vi "ER2007 System Setup Panel.vi"() -> ()   [LabVIEW 2013]
uses:
  Controls/Global ER2007.vi
panel:
  in  "VPA Period":dbl=60.0 caption="(secs)" min=1.0
  in  "Log CGD Errors":bool
  in  "Barometric\nPressure":dbl=14.0 caption="(psig)" min=0.1 step=1.0 format="%.1f"
  in  "SimGalil":bool
  in  "Cell Names":string[](array[string])
  in  "PC ID":i32=1 min=1 max=2
  in  "Excel Template Path":path
  in  "NAII 2250\nWait":dbl=2.0 caption="(sec)" min=0.1 step=1.0 format="%.1f"
  in  "Generator\nON Wait":dbl=3.0 caption="(sec)" min=0.1 step=1.0 format="%.1f"
  in  "Path for Spreadsheet Files":path
  in  "Find Series Resistor\nLow Threshold Level":dbl=25.0 caption="(%)" min=0.1 format="%.1f"
  in  "PrintResData":bool
  in  "Series Resistor\nValues (Kohm)":dbl[](array[numeric])=[0.01, 0.1, 1.0, 10.0, 100.0, 1000.0]
  in  "Series Resistor High\nThreshold Level":dbl=95.0 caption="(%)" min=0.1 format="%.1f"
  in  "Series Resistor Low\nThreshold Level":dbl=10.0 caption="(%)" min=0.1 format="%.1f"
  in  "No File":bool
  in  "Agilent 33220A\nDefault Amplitude":dbl=1.0 caption="(Vrms)" min=0.1 format="%.1f"
  in  "NAII Address":string="02"
  in  "Agilent Address":string="10"
  in  "Super Password":string
  in  "User Password":string
  in  "Data File Path":path
  in  "Graph Update\nInterval":dbl=1.0 caption="(sec)" min=0.1 step=1.0 format="%.1f"
  in  "Calibration Filename":path
  in  "InvDins":bool
  in  "InvDouts":bool
  in  "SimHP":bool
  in  "SimNAI":bool
  in  "Debug":bool
  in  "Quit2LV":bool
  in  "SimDaq":bool
  out "Copyright":string="Program ER2006, Version 1.00, DCI Inc, Copyright 2006, All Rights Reserved"
  in  "Cancel":bool
  in  "OK":bool
  out "Defaults Filename":string="ER2006.dft"
  # "ER2007 System Setup Panel"
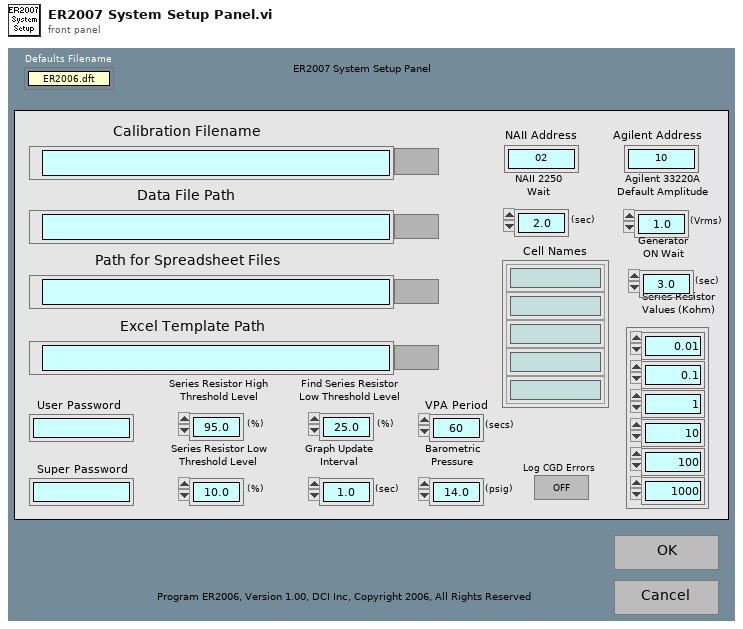
[diagram p1: front panel]
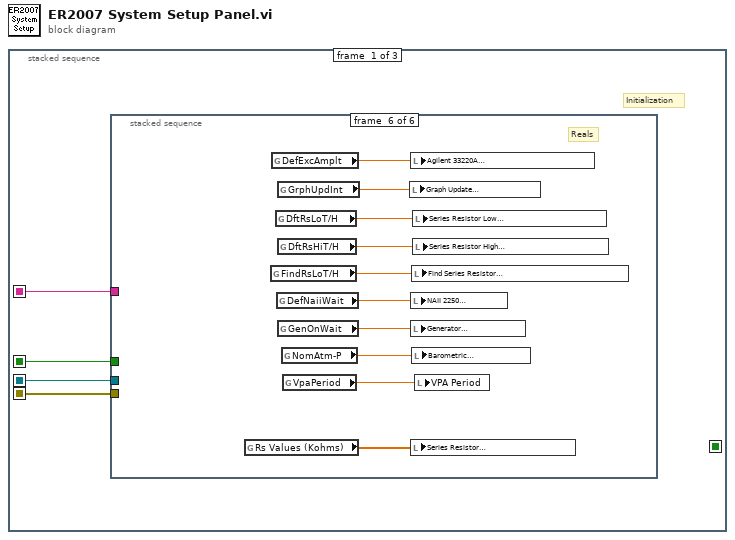
[diagram p0: block diagram]
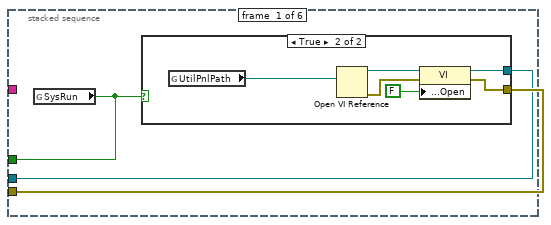
[diagram p2: hidden frame]
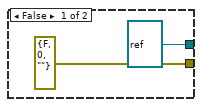
[diagram p3: hidden frame]
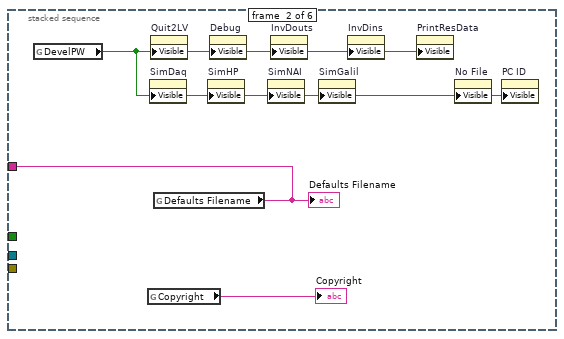
[diagram p4: hidden frame]
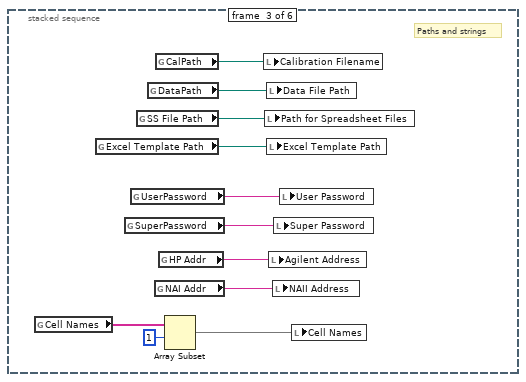
[diagram p5: hidden frame]
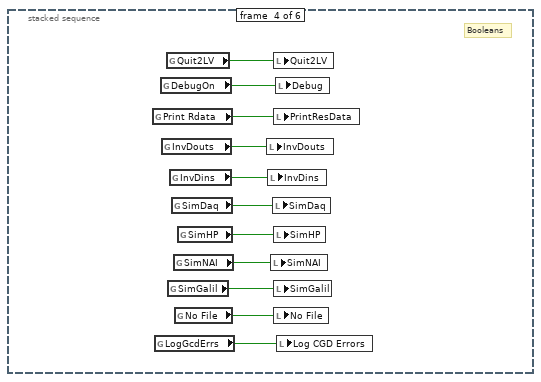
[diagram p6: hidden frame]
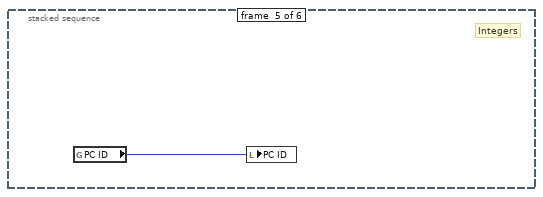
[diagram p7: hidden frame]
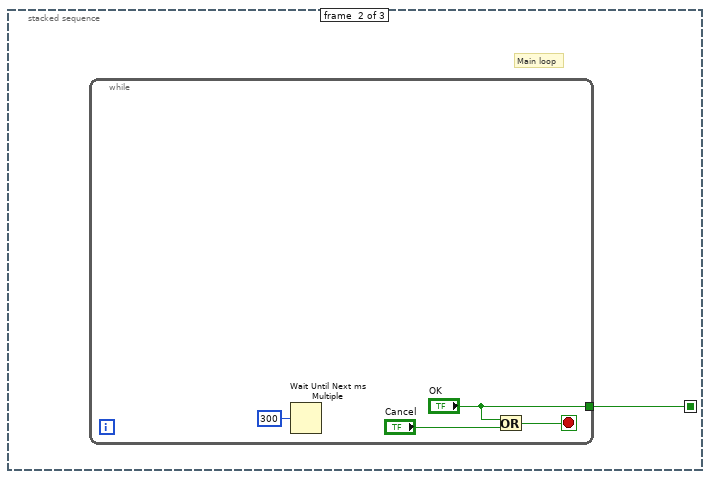
[diagram p8: hidden frame]
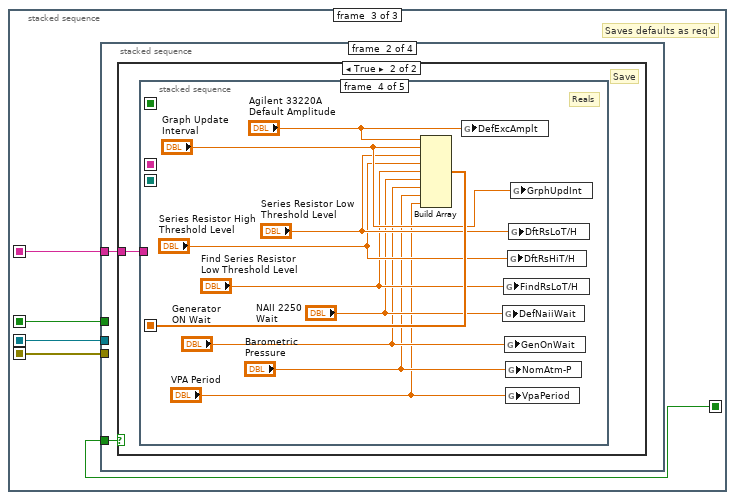
[diagram p9: hidden frame]
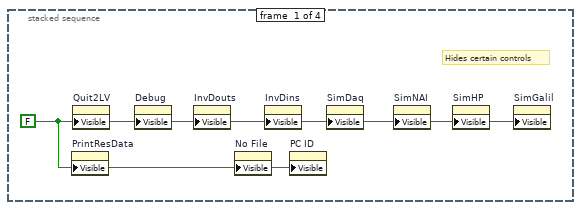
[diagram p10: hidden frame]
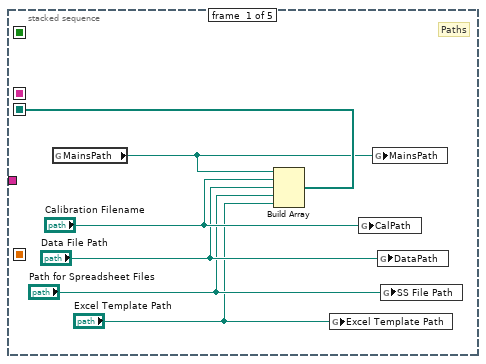
[diagram p12: hidden frame]
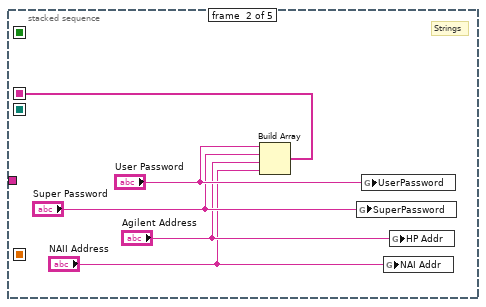
[diagram p13: hidden frame]
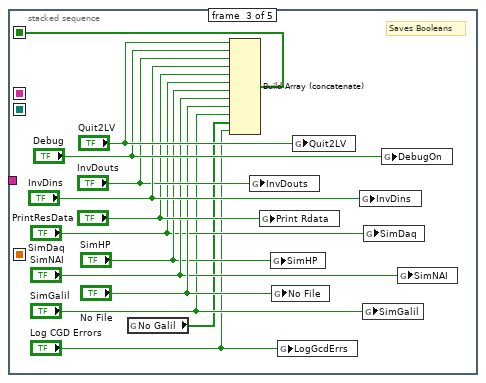
[diagram p14: hidden frame]
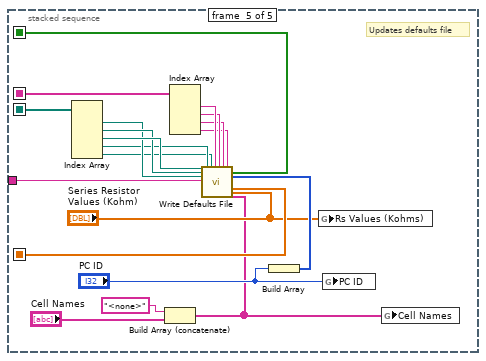
[diagram p15: hidden frame]
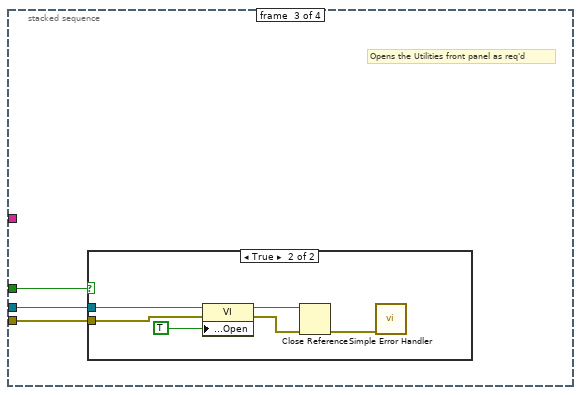
[diagram p16: hidden frame]
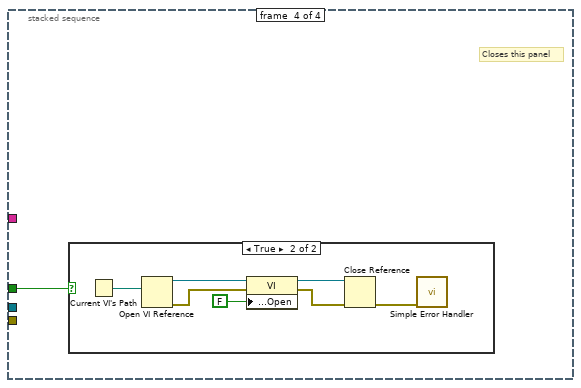
[diagram p18: hidden frame]
diagram:
  n1 = stacked-sequence {
    seq-local: [_ w52 _] -> [_ _ w61]
    seq-local: [w4 _ _] -> [_ _ w60]
    seq-local: [w3 _ _] -> [_ _ w59]
    seq-local: [w1 _ _] -> [_ _ w58]
    seq-local: [w2 _ _] -> [_ _ w57]
    frame #0 {
      # "Initialization"
      n2 = stacked-sequence {
        tunnel: [_ w18 _ _ _ _] -> w4
        tunnel: [w5 _ _ _ _ _] -> w3
        tunnel: [w7 _ _ _ _ _] -> w2
        tunnel: [w6 _ _ _ _ _] -> w1
        frame #0 {
          n3 = global read "Global ER2007.vi" "SysRun"() -> (w5:bool)
          n4 = case shown="True" w5 {
            tunnel: [refnum<vi> refnum w12] -> w6
            tunnel: [errorcluster {"status"=FALSE, "code"=0, "source"=""} ("error out") w11] -> w7
            frame False {
            }
            frame True {
              n5 = global read "Global ER2007.vi" "UtilPnlPath"() -> (w10:path)
              n6 = Open VI Reference(vi path=w10) -> (vi reference=w15:refnum<vi>, error out=w14:errorcluster)  [unwired: 5 in]
              n7 = property class="VI"(reference=w15, error in=w14, "Front Panel Window:Open"=FALSE) -> (reference out=w12:refnum<vi>, error out=w11:errorcluster)
            }
          }
        }
        frame #1 {
          n8 = global read "Global ER2007.vi" "DevelPW"() -> (w16:bool)
          n9 = global read "Global ER2007.vi" "Copyright"() -> (→"Copyright":string)
          n10 = property on="SimDaq" class="Bool (strict)"("Visible"=w16) -> ()  [unwired: 2 in, 2 out]
          n11 = property on="Quit2LV" class="Bool (strict)"("Visible"=w16) -> ()  [unwired: 2 in, 2 out]
          n12 = global read "Global ER2007.vi" "Defaults Filename"() -> (w18:string)
          "Defaults Filename" <- w18
          n13 = property on="SimHP" class="Bool (strict)"("Visible"=w16) -> ()  [unwired: 2 in, 2 out]
          n14 = property on="Debug" class="Bool (strict)"("Visible"=w16) -> ()  [unwired: 2 in, 2 out]
          n15 = property on="SimNAI" class="Bool (strict)"("Visible"=w16) -> ()  [unwired: 2 in, 2 out]
          n16 = property on="InvDouts" class="Bool (strict)"("Visible"=w16) -> ()  [unwired: 2 in, 2 out]
          n17 = property on="SimGalil" class="Bool (strict)"("Visible"=w16) -> ()  [unwired: 2 in, 2 out]
          n18 = property on="InvDins" class="Bool (strict)"("Visible"=w16) -> ()  [unwired: 2 in, 2 out]
          n19 = property on="PrintResData" class="Bool (strict)"("Visible"=w16) -> ()  [unwired: 2 in, 2 out]
          n20 = property on="No File" class="Bool (strict)"("Visible"=w16) -> ()  [unwired: 2 in, 2 out]
          n21 = property on="PC ID" class="DigNum (strict)"("Visible"=w16) -> ()  [unwired: 2 in, 2 out]
        }
        frame #2 {
          # "Paths and strings"
          n22 = global read "Global ER2007.vi" "Cell Names"() -> (w21:string[])
          n23 = global read "Global ER2007.vi" "Excel Template Path"() -> (w26:path)
          n24 = global read "Global ER2007.vi" "SuperPassword"() -> (w24:string)
          n25 = global read "Global ER2007.vi" "UserPassword"() -> (w25:string)
          n26 = global read "Global ER2007.vi" "SS File Path"() -> (w27:path)
          n27 = global read "Global ER2007.vi" "DataPath"() -> (w28:path)
          n28 = global read "Global ER2007.vi" "NAI Addr"() -> (w22:string)
          n29 = global read "Global ER2007.vi" "CalPath"() -> (w29:path)
          n30 = global read "Global ER2007.vi" "HP Addr"() -> (w23:string)
          n31 = Array Subset(array=w21, index=1) -> (w19:string[])  [unwired: 1 in]
          n32 = local write "Calibration Filename"(w29) -> ()
          n33 = local write "Path for Spreadsheet Files"(w27) -> ()
          n34 = local write "Data File Path"(w28) -> ()
          n35 = local write "Excel Template Path"(w26) -> ()
          n36 = local write "Agilent Address"(w23) -> ()
          n37 = local write "NAII Address"(w22) -> ()
          n38 = local write "Super Password"(w24) -> ()
          n39 = local write "User Password"(w25) -> ()
          n40 = local write "Cell Names"(w19) -> ()
        }
        frame #3 {
          # "Booleans"
          n41 = global read "Global ER2007.vi" "Print Rdata"() -> (w38:bool)
          n42 = global read "Global ER2007.vi" "LogGcdErrs"() -> (w30:bool)
          n43 = global read "Global ER2007.vi" "DebugOn"() -> (w39:bool)
          n44 = global read "Global ER2007.vi" "InvDouts"() -> (w37:bool)
          n45 = global read "Global ER2007.vi" "Quit2LV"() -> (w40:bool)
          n46 = global read "Global ER2007.vi" "SimGalil"() -> (w31:bool)
          n47 = global read "Global ER2007.vi" "InvDins"() -> (w36:bool)
          n48 = global read "Global ER2007.vi" "SimDaq"() -> (w35:bool)
          n49 = global read "Global ER2007.vi" "SimNAI"() -> (w33:bool)
          n50 = global read "Global ER2007.vi" "No File"() -> (w32:bool)
          n51 = global read "Global ER2007.vi" "SimHP"() -> (w34:bool)
          n52 = local write "InvDouts"(w37) -> ()
          n53 = local write "InvDins"(w36) -> ()
          n54 = local write "SimNAI"(w33) -> ()
          n55 = local write "SimDaq"(w35) -> ()
          n56 = local write "Quit2LV"(w40) -> ()
          n57 = local write "PrintResData"(w38) -> ()
          n58 = local write "SimHP"(w34) -> ()
          n59 = local write "SimGalil"(w31) -> ()
          n60 = local write "No File"(w32) -> ()
          n61 = local write "Debug"(w39) -> ()
          n62 = local write "Log CGD Errors"(w30) -> ()
        }
        frame #4 {
          # "Integers"
          n63 = global read "Global ER2007.vi" "PC ID"() -> (w41:i32)
          n64 = local write "PC ID"(w41) -> ()
        }
        frame #5 {
          # "Reals"
          n65 = global read "Global ER2007.vi" "Rs Values (Kohms)"() -> (w44:dbl[])
          n66 = global read "Global ER2007.vi" "FindRsLoT/H"() -> (w47:dbl)
          n67 = global read "Global ER2007.vi" "DefExcAmplt"() -> (w51:dbl)
          n68 = global read "Global ER2007.vi" "DftRsLoT/H"() -> (w49:dbl)
          n69 = global read "Global ER2007.vi" "DefNaiiWait"() -> (w46:dbl)
          n70 = global read "Global ER2007.vi" "GrphUpdInt"() -> (w50:dbl)
          n71 = global read "Global ER2007.vi" "DftRsHiT/H"() -> (w48:dbl)
          n72 = global read "Global ER2007.vi" "GenOnWait"() -> (w45:dbl)
          n73 = global read "Global ER2007.vi" "NomAtm-P"() -> (w43:dbl)
          n74 = global read "Global ER2007.vi" "VpaPeriod"() -> (w42:dbl)
          n75 = local write "Graph Update\nInterval"(w50) -> ()
          n76 = local write "Agilent 33220A\nDefault Amplitude"(w51) -> ()
          n77 = local write "NAII 2250\nWait"(w46) -> ()
          n78 = local write "Generator\nON Wait"(w45) -> ()
          n79 = local write "Series Resistor\nValues (Kohm)"(w44) -> ()
          n80 = local write "Find Series Resistor\nLow Threshold Level"(w47) -> ()
          n81 = local write "Barometric\nPressure"(w43) -> ()
          n82 = local write "Series Resistor Low\nThreshold Level"(w49) -> ()
          n83 = local write "Series Resistor High\nThreshold Level"(w48) -> ()
          n84 = local write "VPA Period"(w42) -> ()
        }
      }
    }
    frame #1 {
      # "Main loop"
      n85 = while {
        tunnel: ["OK"] -> w52
        stop <- w55 stop-if-true
        n86 = Wait Until Next ms Multiple(millisecond multiple=u32 300) -> ()  [unwired: 1 out]
        n87 = Or(x="OK", y="Cancel") -> (x .or. y?=w55:bool)
      }
    }
    frame #2 {
      # "Saves defaults as req'd"
      n88 = stacked-sequence {
        tunnel: w61 -> [_ w64 _ _]
        tunnel: w60 -> [_ w63 _ _]
        tunnel: w59 -> [_ _ w122 w129]
        tunnel: w58 -> [_ _ w121 _]
        tunnel: w57 -> [_ _ w120 _]
        frame #0 {
          w62 = FALSE ("Visible")
          # "Hides certain controls"
          n89 = property on="PrintResData" class="Bool (strict)"("Visible"=w62) -> ()  [unwired: 2 in, 2 out]
          n90 = property on="Quit2LV" class="Bool (strict)"("Visible"=w62) -> ()  [unwired: 2 in, 2 out]
          n91 = property on="Debug" class="Bool (strict)"("Visible"=w62) -> ()  [unwired: 2 in, 2 out]
          n92 = property on="InvDouts" class="Bool (strict)"("Visible"=w62) -> ()  [unwired: 2 in, 2 out]
          n93 = property on="No File" class="Bool (strict)"("Visible"=w62) -> ()  [unwired: 2 in, 2 out]
          n94 = property on="InvDins" class="Bool (strict)"("Visible"=w62) -> ()  [unwired: 2 in, 2 out]
          n95 = property on="PC ID" class="DigNum (strict)"("Visible"=w62) -> ()  [unwired: 2 in, 2 out]
          n96 = property on="SimDaq" class="Bool (strict)"("Visible"=w62) -> ()  [unwired: 2 in, 2 out]
          n97 = property on="SimNAI" class="Bool (strict)"("Visible"=w62) -> ()  [unwired: 2 in, 2 out]
          n98 = property on="SimHP" class="Bool (strict)"("Visible"=w62) -> ()  [unwired: 2 in, 2 out]
          n99 = property on="SimGalil" class="Bool (strict)"("Visible"=w62) -> ()  [unwired: 2 in, 2 out]
        }
        frame #1 {
          n100 = case shown="True" w64 {
            tunnel: w63 -> [_ w65]
            frame False {
            }
            frame True {
              # "Save"
              n101 = stacked-sequence {
                seq-local: [_ _ w89 _ _] -> [_ _ _ _ w118]
                seq-local: [w71 _ _ _ _] -> [_ _ _ _ w117]
                seq-local: [_ w76 _ _ _] -> [_ _ _ _ w113]
                seq-local: [_ _ _ w99 _] -> [_ _ _ _ w108]
                tunnel: w65 -> [_ _ _ _ w119]
                frame #0 {
                  # "Paths"
                  n102 = global read "Global ER2007.vi" "MainsPath"() -> (w70:path)
                  n103 = Build Array(w70, "Calibration Filename", "Data File Path", "Path for Spreadsheet Files", "Excel Template Path") -> (w71:path[])
                  n104 = global write "Global ER2007.vi" "Excel Template Path"("Excel Template Path") -> ()
                  n105 = global write "Global ER2007.vi" "CalPath"("Calibration Filename") -> ()
                  n106 = global write "Global ER2007.vi" "MainsPath"(w70) -> ()
                  n107 = global write "Global ER2007.vi" "DataPath"("Data File Path") -> ()
                  n108 = global write "Global ER2007.vi" "SS File Path"("Path for Spreadsheet Files") -> ()
                }
                frame #1 {
                  # "Strings"
                  n109 = Build Array("User Password", "Super Password", "Agilent Address", "NAII Address") -> (w76:string[])
                  n110 = global write "Global ER2007.vi" "SuperPassword"("Super Password") -> ()
                  n111 = global write "Global ER2007.vi" "UserPassword"("User Password") -> ()
                  n112 = global write "Global ER2007.vi" "NAI Addr"("NAII Address") -> ()
                  n113 = global write "Global ER2007.vi" "HP Addr"("Agilent Address") -> ()
                }
                frame #2 {
                  # "Saves Booleans"
                  n114 = global read "Global ER2007.vi" "No Galil"() -> (w78:bool[])
                  n115 = Build Array (concatenate)("Quit2LV", "Debug", "InvDouts", "InvDins", "PrintResData", "SimDaq", "SimHP", "SimNAI", "No File", "SimGalil", w78, "Log CGD Errors") -> (w89:bool[])
                  n116 = global write "Global ER2007.vi" "InvDouts"("InvDouts") -> ()
                  n117 = global write "Global ER2007.vi" "Print Rdata"("PrintResData") -> ()
                  n118 = global write "Global ER2007.vi" "SimHP"("SimHP") -> ()
                  n119 = global write "Global ER2007.vi" "No File"("No File") -> ()
                  n120 = global write "Global ER2007.vi" "LogGcdErrs"("Log CGD Errors") -> ()
                  n121 = global write "Global ER2007.vi" "Quit2LV"("Quit2LV") -> ()
                  n122 = global write "Global ER2007.vi" "InvDins"("InvDins") -> ()
                  n123 = global write "Global ER2007.vi" "SimGalil"("SimGalil") -> ()
                  n124 = global write "Global ER2007.vi" "SimDaq"("SimDaq") -> ()
                  n125 = global write "Global ER2007.vi" "DebugOn"("Debug") -> ()
                  n126 = global write "Global ER2007.vi" "SimNAI"("SimNAI") -> ()
                }
                frame #3 {
                  # "Reals"
                  n127 = Build Array("Agilent 33220A\nDefault Amplitude", "Graph Update\nInterval", "Series Resistor Low\nThreshold Level", "Series Resistor High\nThreshold Level", "Find Series Resistor\nLow Threshold Level", "NAII 2250\nWait", "Generator\nON Wait", "Barometric\nPressure", "VPA Period") -> (w99:dbl[])
                  n128 = global write "Global ER2007.vi" "DefExcAmplt"("Agilent 33220A\nDefault Amplitude") -> ()
                  n129 = global write "Global ER2007.vi" "DefNaiiWait"("NAII 2250\nWait") -> ()
                  n130 = global write "Global ER2007.vi" "FindRsLoT/H"("Find Series Resistor\nLow Threshold Level") -> ()
                  n131 = global write "Global ER2007.vi" "GenOnWait"("Generator\nON Wait") -> ()
                  n132 = global write "Global ER2007.vi" "NomAtm-P"("Barometric\nPressure") -> ()
                  n133 = global write "Global ER2007.vi" "VpaPeriod"("VPA Period") -> ()
                  n134 = global write "Global ER2007.vi" "DftRsHiT/H"("Series Resistor High\nThreshold Level") -> ()
                  n135 = global write "Global ER2007.vi" "DftRsLoT/H"("Series Resistor Low\nThreshold Level") -> ()
                  n136 = global write "Global ER2007.vi" "GrphUpdInt"("Graph Update\nInterval") -> ()
                }
                frame #4 {
                  # "Updates defaults file"
                  n137 = Index Array(array=w117) -> (element #1=w114:path, element #2=w115:path, element #3=w116:path, element #4=w107:path, element #5=w106:path)  [unwired: 5 in]
                  n138 = Build Array (concatenate)("<none>", "Cell Names") -> (w100:string[])
                  n139 = Index Array(array=w113) -> (element #1=w112:string, element #2=w111:string, element #3=w110:string, element #4=w109:string)  [unwired: 4 in]
                  n140 = Build Array("PC ID") -> (w105:i32[])
                  n141 = call "Write Defaults File.vi"("DirPath3"=w116, "DirPath2"=w115, "DirPath1"=w114, "DefaultFilename"=w119, "DirPath4"=w107, "DirPath5"=w106, "String1"=w112, "String2"=w111, "String3"=w110, "String4"=w109, "BooleanArray"=w118, "IntegerArray1"=w105, "RealArray1"=w108, "RealArray2"="Series Resistor\nValues (Kohm)", "StringArray"=w100) -> ()  [unwired: 13 in]
                  n142 = global write "Global ER2007.vi" "Rs Values (Kohms)"("Series Resistor\nValues (Kohm)") -> ()
                  n143 = global write "Global ER2007.vi" "PC ID"("PC ID") -> ()
                  n144 = global write "Global ER2007.vi" "Cell Names"(w100) -> ()
                }
              }
            }
          }
        }
        frame #2 {
          # "Opens the Utilities front panel as req'd"
          n145 = case shown="True" w122 {
            tunnel: w121 -> [_ w128]
            tunnel: w120 -> [_ w127]
            frame False {
              # "Not a System run"
            }
            frame True {
              n146 = property class="VI"(reference=w128, error in=w127, "Front Panel Window:Open"=TRUE) -> (reference out=w125:refnum<vi>, error out=w124:errorcluster)
              n147 = Close Reference(reference=w125, error in (no error)=w124) -> (error out=w123:errorcluster)
              n148 = call <vilib>:"Simple Error Handler.vi"("error in (no error)"=w123) -> ()  [unwired: 4 in, 5 out]
            }
          }
        }
        frame #3 {
          # "Closes this panel"
          n149 = case shown="True" w129 {
            frame False {
            }
            frame True {
              n150 = Current VI's Path() -> (path=w136:path)
              n151 = Open VI Reference(vi path=w136) -> (vi reference=w135:refnum<vi>, error out=w134:errorcluster)  [unwired: 5 in]
              n152 = property class="VI"(reference=w135, error in=w134, "Front Panel Window:Open"=FALSE) -> (reference out=w132:refnum<vi>, error out=w131:errorcluster)
              n153 = Close Reference(reference=w132, error in (no error)=w131) -> (error out=w130:errorcluster)
              n154 = call <vilib>:"Simple Error Handler.vi"("error in (no error)"=w130) -> ()  [unwired: 4 in, 5 out]
            }
          }
        }
      }
    }
  }
